vi "Write Peasant Attributes.vi"(8 "error in (no error)":errorcluster, 10 "Peasant":T1, 11 "Peasant in":refnum<class "Peasant.lvclass">) -> (0 "error out":errorcluster, 3 "Peasant out":refnum<class "Peasant.lvclass">)   [LabVIEW 2021, in "Peasant.lvclass"]
uses:
  Peasant.lvclass
  PeasantAttributes.ctl
  Peasant.lvclass/Peasant.ctl
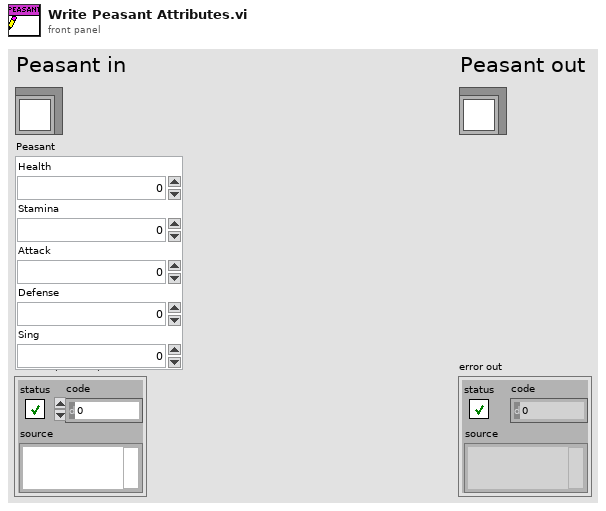
[diagram p1: front panel]
types:
  T1 = typedef "Peasant.lvclass/PeasantAttributes.ctl" = cluster{"Health":i32, "Stamina":i32, "Attack":i32, "Defense":i32, "Sing":i32}
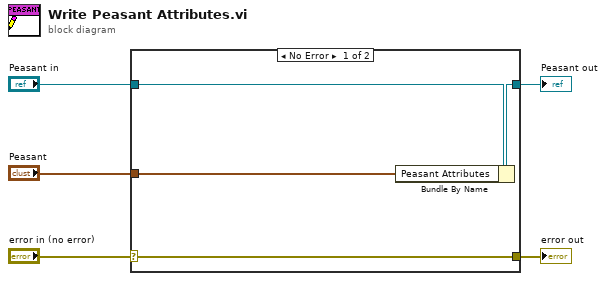
[diagram p0: block diagram]
diagram:
  n1 = case shown="No Error" "error in (no error)" {
    selector: "error in (no error)" -> [w9 w10]
    tunnel: [w9 w10] -> w4
    tunnel: [w7 w11] -> w2
    tunnel: "Peasant in" -> [w8 w11]
    tunnel: "Peasant" -> [w6 _]
    frame No Error {
      n2 = Bundle By Name(cluster=w8, "Peasant Attributes"=w6) -> (w7:refnum<class "Peasant.lvclass">)
    }
    frame Error {
    }
  }
  "error out" <- w4
  "Peasant out" <- w2
